vi "Async Worker.vi"(8 "error in (no error)":errorcluster, 10 "Events":T1, 11 "Controller Ref":refnum<k1>) -> (0 "error out":errorcluster, 2 "button info":T2, 3 "Refnum out":refnum<k1>)   [LabVIEW 2011, in "LVH-Xbox-One-Controller.lvlib"]
uses:
  LVH-Xbox-One-Controller.lvlib
  <vilib>/Utility/inputDevices.llb/joystickAcquire.vi
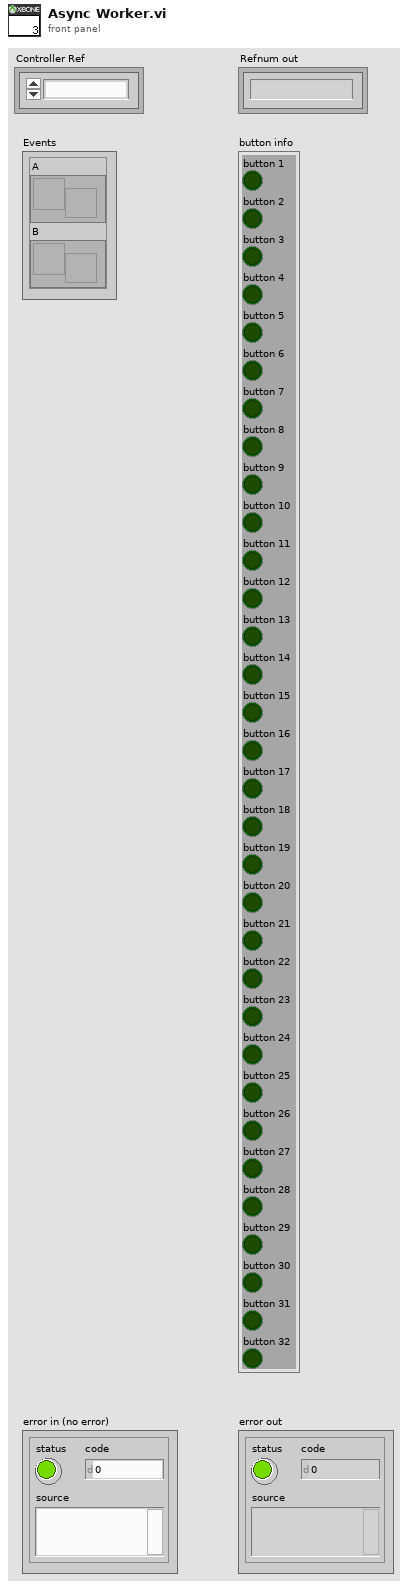
[diagram p1: front panel]
types:
  T1 = cluster{"A":refnum<user-event>, "B":refnum<user-event>}
  T2 = cluster{"button 1":bool, "button 2":bool, "button 3":bool, "button 4":bool, "button 5":bool, "button 6":bool, "button 7":bool, "button 8":bool, "button 9":bool, "button 10":bool, "button 11":bool, "button 12":bool, "button 13":bool, "button 14":bool, "button 15":bool, "button 16":bool, "button 17":bool, "button 18":bool, "button 19":bool, "button 20":bool, "button 21":bool, "button 22":bool, "button 23":bool, "button 24":bool, "button 25":bool, "button 26":bool, "button 27":bool, "button 28":bool, "button 29":bool, "button 30":bool, "button 31":bool, "button 32":bool}
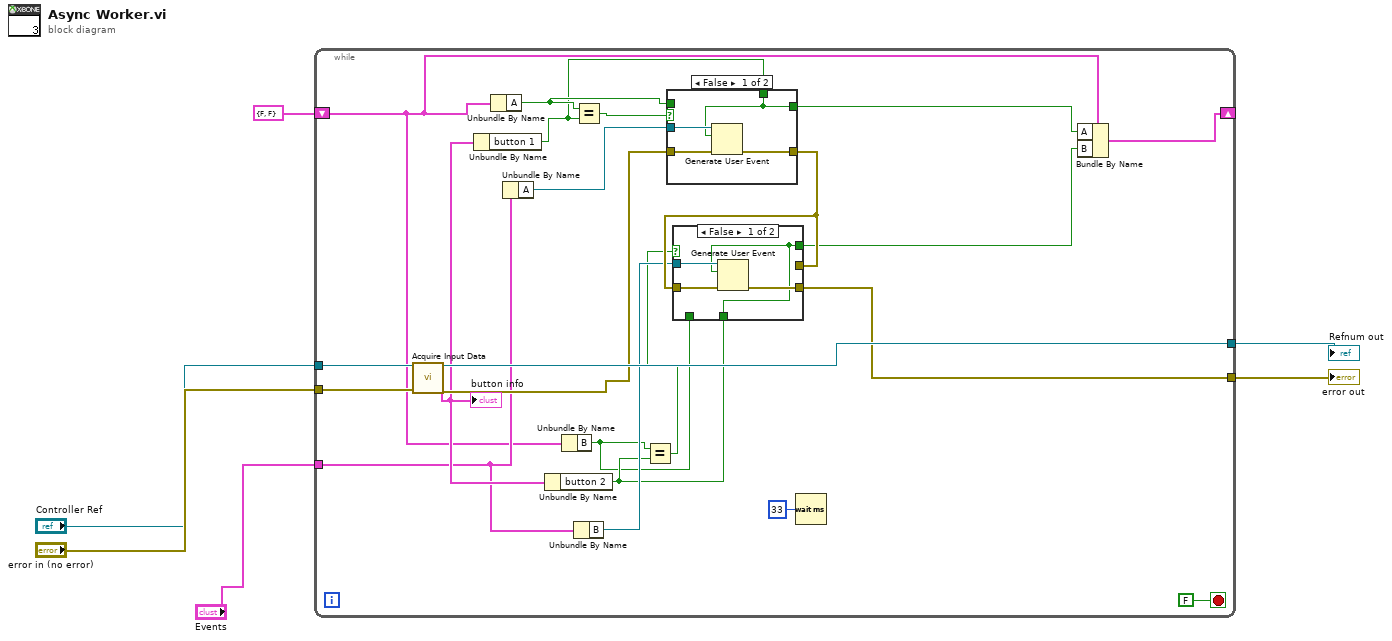
[diagram p0: block diagram]
diagram:
  n1 = while {
    tunnel: [w28] -> w1
    tunnel: [w20] -> w2
    tunnel: "Controller Ref" -> [w27]
    tunnel: "error in (no error)" -> [w26]
    tunnel: "Events" -> [w21]
    shift-right: [w9] -> _
    shift-left: cluster{"A":bool, "B":bool} {"A"=FALSE, "B"=FALSE} -> [w16]
    stop <- FALSE stop-if-true
    n2 = call-poly <vilib>:"Acquire Input Data.vi"("device ID"=w27, "error in (no error)"=w26) -> ("device ID"=w28:refnum<k1>, "button info"=w22:T2, "error out"=w24:errorcluster)  [unwired: 13 in, 2 out]
    "button info" <- w22
    n3 = Unbundle By Name(w22) -> ("button 1"=w13:bool)
    n4 = Unbundle By Name(w16) -> ("A"=w14:bool)
    n5 = Unbundle By Name(w21) -> ("A"=w23:refnum<user-event>)
    n6 = Unbundle By Name(w22) -> ("button 2"=w11:bool)
    n7 = Unbundle By Name(w16) -> ("B"=w10:bool)
    n8 = Equal?(x=w14, y=w13) -> (x = y?=w25:bool)
    n9 = Unbundle By Name(w21) -> ("B"=w18:refnum<user-event>)
    n10 = Equal?(x=w10, y=w11) -> (x = y?=w17:bool)
    n11 = case shown="False" w25 {
      tunnel: w24 -> [w38 w40]
      tunnel: [w37 w40] -> w19
      tunnel: w23 -> [w36 _]
      tunnel: [w35 w39] -> w15
      tunnel: w14 -> [_ w39]
      tunnel: w13 -> [w35 _]
      frame False {
        n12 = Generate User Event(user event=w36, event data cluster=w35, error in=w38) -> (error out=w37:errorcluster)  [unwired: 1 out]
      }
      frame True {
        # "No Change"
      }
    }
    n13 = case shown="False" w17 {
      tunnel: w19 -> [w32 w34]
      tunnel: [w31 w34] -> w20
      tunnel: w18 -> [w30 _]
      tunnel: w19 -> [_ _]
      tunnel: [w29 w33] -> w12
      tunnel: w11 -> [w29 _]
      tunnel: w10 -> [_ w33]
      frame False {
        n14 = Generate User Event(user event=w30, event data cluster=w29, error in=w32) -> (error out=w31:errorcluster)  [unwired: 1 out]
      }
      frame True {
        # "No Change"
      }
    }
    n15 = Wait (ms)(milliseconds to wait=u32 33) -> ()  [unwired: 1 out]
    n16 = Bundle By Name(cluster=w16, "A"=w15, "B"=w12) -> (w9:cluster{"A":bool, "B":bool})
  }
  "error out" <- w2
  "Refnum out" <- w1
